vi "GD Status.vi"() -> (1 "Error":T1, 2 "Störung":bool, 3 "Status":string)   [LabVIEW 2020, in "EPA 1065.lvlib" / "HovaCAL Interference verificaton.lvlib"]
uses:
  HovaCAL Interference verificaton.lvlib
  Linearisierung V2/Gasteiler/AK-Komm Gasteiler/Aktionen AK Komm.ctl
  Linearisierung V2/Gasteiler/AK-Komm Gasteiler/AK Komm Gasteiler.lvlib
  Linearisierung V2/Aktion FGV Stoerungen sammeln und auswerten.ctl
  Linearisierung V2/Linearisierung v2.lvlib
  Linearisierung V2/Gasteiler/AK-Komm Gasteiler/Alter Gasteiler/Aktionen AK Komm_ALT.ctl
  Linearisierung V2/Gasteiler/AK-Komm Gasteiler/Alter Gasteiler/Alter Gasteiler.lvlib
  Linearisierung V2/Gasteiler/Horiba/Aktion Befehl.ctl
  Linearisierung V2/Gasteiler/Horiba/Horiba GDC.lvlib
  Linearisierung V2/Gasteiler/HovaCAL_Interface/Kommunikation/Aktion_FGV_HovaCAL_Interface_Kommandos.ctl
  Linearisierung V2/Gasteiler/HovaCAL_Interface/Kommunikation/Kommunikation.lvlib
  Linearisierung V2/Gasteiler/Aktionen FGV Gasteiler Daten.ctl
  Linearisierung V2/Gasteiler/Gasteiler.lvlib
  Linearisierung V2/Gasteiler/Gasteiler Fehler.ctl
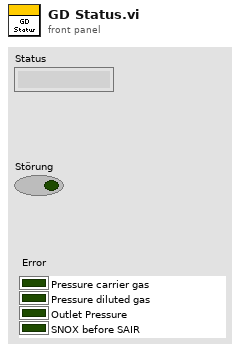
[diagram p1: front panel]
types:
  T1 = typedef "Linearisierung v2.lvlib/Gasteiler.lvlib/Gasteiler Fehler.ctl" = cluster{"Pressure carrier gas":bool, "Pressure diluted gas":bool, "Outlet Pressure":bool, "SNOX before SAIR":bool}
  T2 = typedef "Linearisierung v2.lvlib/Gasteiler.lvlib/Aktionen FGV Gasteiler Daten.ctl" = enum16{"lesen", "Gasteiler Daten", "Seriellen Param.", "MB-Endwert", "laden", "speichern", "Anforderung", "TCP", "Aufzeichnung Start"}
  T3 = typedef "Linearisierung v2.lvlib/GasteilerType.ctl" = u16
  T4 = typedef "Linearisierung v2.lvlib/Aktion FGV Stoerungen sammeln und auswerten.ctl" = enum16{"init", "lesen", "error", "prüfen", "reset error", "abbrechen", "fortsetzen", "neustart", "Bedientasten reset"}
  T5 = typedef "Linearisierung v2.lvlib/Gasteiler.lvlib/AK Komm Gasteiler.lvlib/Aktionen AK Komm.ctl" = enum16{"lesen", "initialisieren", "beenden", "Status", "SMAN", "SREM", "STBY", "ASTF", "ASTZ", "SLST", "AGAT", "EGAK", "AGAK", "AKAK", "ADRU", "SKOP", "SVSA", "SVSZ", "SONO", "SAIR", "SNOX", "ANOX", "SSPL", "SRUC", "SLIN", "ALST", "ETYP", "SVIO", "LCYL", "CCYL", "DCYL", "SCYL", "GCYL", "DRGV", "DRDC"}
  T6 = typedef "Linearisierung v2.lvlib/Gasteiler.lvlib/AK Komm Gasteiler.lvlib/Alter Gasteiler.lvlib/Aktionen AK Komm_ALT.ctl" = enum16{"lesen", "initialisieren", "beenden", "SRES", "STBY", "SREM", "SMAN", "SLIN", "SLCH", "SLST", "SSPL", "AGAT", "ALST", "ASTZ", "ASTF", "AGAK", "EGAK"}
  T7 = typedef "Linearisierung v2.lvlib/Gasteiler.lvlib/Horiba GDC.lvlib/Aktion Befehl.ctl" = enum16{"lesen", "initialisieren", "Beenden", "Standby", "GD/CC", "Info", "Flow", "Alarm", "GD parameter", "GD point", "Durchfluss", "Spuelen1", "Spuelen1 On", "Spuelen1Off", "Spuelen2", "Ventil-Abfrage", "Reset"}
  T8 = typedef "Linearisierung v2.lvlib/Gasteiler.lvlib/HovaCAL_Interface.lvlib/Kommunikation.lvlib/Aktion_FGV_HovaCAL_Interface_Kommandos.ctl" = enum16{"lesen", "verarbeiten", "hinzufügen", "on top", "init", "sammeln", "freigeben", "connected"}
  T9 = typedef "Linearisierung v2.lvlib/LIN ErrorCluster.ctl" = cluster{"Störung Kommunikation":bool, "Pressure carrier gas":bool, "Pressure diluted gas":bool, "Outlet Pressure":bool, "SNOX before SAIR":bool, "Störung Gasteiler":bool}
  T10 = cluster{"Pressure carrier gas":bool, "Pressure diluted gas":bool, "Outlet Pressure":bool, bool}
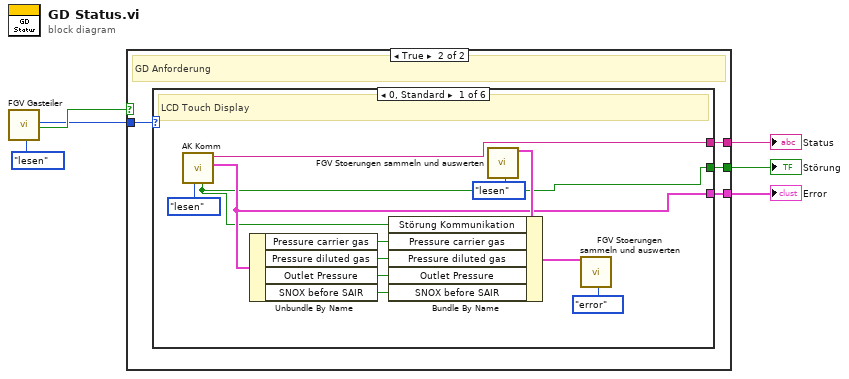
[diagram p0: block diagram]
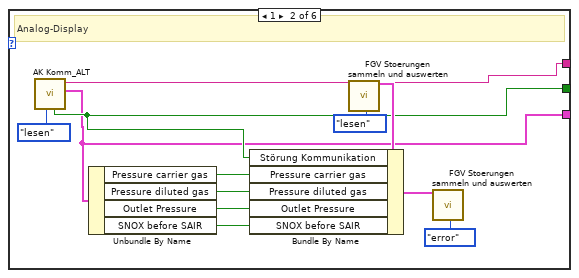
[diagram p3: hidden frame]
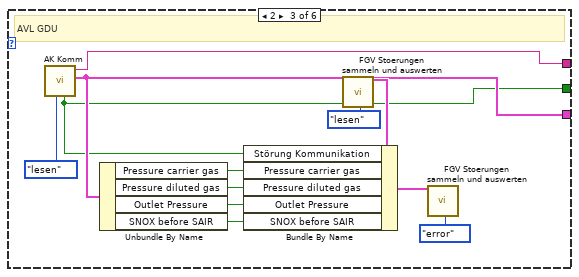
[diagram p4: hidden frame]
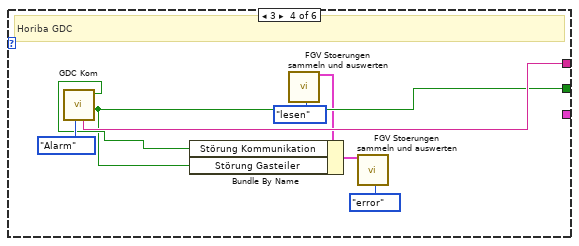
[diagram p5: hidden frame]
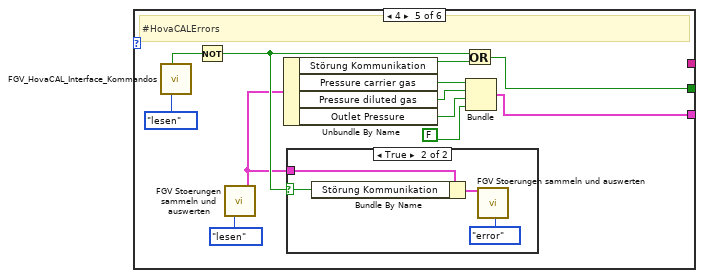
[diagram p6: hidden frame]
diagram:
  n1 = call "FGV Gasteiler.vi"("Aktionen"=Aktionen_FGV_Gasteiler_Daten."lesen") -> ("Gasteiler Type"=w2:T3, "Anforderung"=w3:bool)  [unwired: 11 in, 6 out]
  n2 = case shown="True" w3 {
    tunnel: w2 -> [_ w10]
    tunnel: [_ w9] -> w4
    tunnel: [_ w8] -> w5
    tunnel: [_ w7] -> w6
    frame False {
    }
    frame True {
      # "GD Anforderung"
      n3 = case shown="0, Standard" w10 {
        tunnel: [w12 w23 w37 _ w56 _] -> w9
        tunnel: [w11 w24 w36 w48 w55 _] -> w8
        tunnel: [w13 w25 w35 w50 _ _] -> w7
        frame 0, Default {
          # "LCD Touch Display"
          n4 = call "AK Komm.vi"("Aktionen"=Aktionen_AK_Komm."lesen") -> ("Error"=w12:T1, "Status"=w13:string, "Störung Kommunikation"=w11:bool)  [unwired: 4 in, 4 out]
          n5 = Unbundle By Name(w12) -> ("Pressure carrier gas"=w18:bool, "Pressure diluted gas"=w17:bool, "Outlet Pressure"=w16:bool, "SNOX before SAIR"=w15:bool)
          n6 = call "FGV Stoerungen sammeln und auswerten.vi"("Aktion"=Aktion_FGV_Stoerungen_sammeln_und_auswerten."lesen") -> ("Errors"=w19:T9)  [unwired: 12 in, 6 out]
          n7 = Bundle By Name(cluster=w19, "Störung Kommunikation"=w11, "Pressure carrier gas"=w18, "Pressure diluted gas"=w17, "Outlet Pressure"=w16, "SNOX before SAIR"=w15) -> (w14:T9)
          n8 = call "FGV Stoerungen sammeln und auswerten.vi"("Errors"=w14, "Aktion"=Aktion_FGV_Stoerungen_sammeln_und_auswerten."error") -> ()  [unwired: 11 in, 7 out]
        }
        frame 1 {
          # "Analog-Display"
          n9 = call "AK Komm_ALT.vi"("Aktionen_ALT"=Aktionen_AK_Komm_ALT."lesen") -> ("Error"=w23:T1, "Status"=w25:string, "Störung Kommunikation"=w24:bool)  [unwired: 6 in, 2 out]
          n10 = Unbundle By Name(w23) -> ("Pressure carrier gas"=w30:bool, "Pressure diluted gas"=w29:bool, "Outlet Pressure"=w28:bool, "SNOX before SAIR"=w27:bool)
          n11 = call "FGV Stoerungen sammeln und auswerten.vi"("Aktion"=Aktion_FGV_Stoerungen_sammeln_und_auswerten."lesen") -> ("Errors"=w31:T9)  [unwired: 12 in, 6 out]
          n12 = Bundle By Name(cluster=w31, "Störung Kommunikation"=w24, "Pressure carrier gas"=w30, "Pressure diluted gas"=w29, "Outlet Pressure"=w28, "SNOX before SAIR"=w27) -> (w26:T9)
          n13 = call "FGV Stoerungen sammeln und auswerten.vi"("Errors"=w26, "Aktion"=Aktion_FGV_Stoerungen_sammeln_und_auswerten."error") -> ()  [unwired: 11 in, 7 out]
        }
        frame 2 {
          # "AVL GDU"
          n14 = call "AK Komm.vi"("Aktionen"=Aktionen_AK_Komm."lesen") -> ("Error"=w37:T1, "Status"=w35:string, "Störung Kommunikation"=w36:bool)  [unwired: 4 in, 4 out]
          n15 = Unbundle By Name(w37) -> ("Pressure carrier gas"=w42:bool, "Pressure diluted gas"=w41:bool, "Outlet Pressure"=w40:bool, "SNOX before SAIR"=w39:bool)
          n16 = call "FGV Stoerungen sammeln und auswerten.vi"("Aktion"=Aktion_FGV_Stoerungen_sammeln_und_auswerten."lesen") -> ("Errors"=w43:T9)  [unwired: 12 in, 6 out]
          n17 = Bundle By Name(cluster=w43, "Störung Kommunikation"=w36, "Pressure carrier gas"=w42, "Pressure diluted gas"=w41, "Outlet Pressure"=w40, "SNOX before SAIR"=w39) -> (w38:T9)
          n18 = call "FGV Stoerungen sammeln und auswerten.vi"("Errors"=w38, "Aktion"=Aktion_FGV_Stoerungen_sammeln_und_auswerten."error") -> ()  [unwired: 11 in, 7 out]
        }
        frame 3 {
          # "Horiba GDC"
          n19 = call "GDC Kom.vi"("Befehl"=Aktion_Befehl."Alarm") -> ("Status (alarm)"=w48:bool, "Fehler"=w49:bool, "Status"=w50:string)  [unwired: 4 in, 4 out]
          n20 = call "FGV Stoerungen sammeln und auswerten.vi"("Aktion"=Aktion_FGV_Stoerungen_sammeln_und_auswerten."lesen") -> ("Errors"=w47:T9)  [unwired: 12 in, 6 out]
          n21 = Bundle By Name(cluster=w47, "Störung Kommunikation"=w49, "Störung Gasteiler"=w48) -> (w51:T9)
          n22 = call "FGV Stoerungen sammeln und auswerten.vi"("Errors"=w51, "Aktion"=Aktion_FGV_Stoerungen_sammeln_und_auswerten."error") -> ()  [unwired: 11 in, 7 out]
        }
        frame 4 {
          # "#HovaCALErrors"
          n23 = call "FGV_HovaCAL_Interface_Kommandos.vi"("Aktion"=Aktion_FGV_HovaCAL_Interface_Kommandos."lesen") -> ("connected out ?"=w58:bool)  [unwired: 4 in, 5 out]
          n24 = Not(x=w58) -> (.not. x?=w59:bool)
          n25 = call "FGV Stoerungen sammeln und auswerten.vi"("Aktion"=Aktion_FGV_Stoerungen_sammeln_und_auswerten."lesen") -> ("Errors for AutoSPAN"=w57:T9)  [unwired: 12 in, 6 out]
          n26 = Unbundle By Name(w57) -> ("Störung Kommunikation"=w65:bool, "Pressure carrier gas"=w64:bool, "Pressure diluted gas"=w63:bool, "Outlet Pressure"=w62:bool)
          n27 = case shown="True" w59 {
            selector: w59 -> [_ w68]
            tunnel: w57 -> [_ w67]
            frame False {
            }
            frame True {
              n28 = Bundle By Name(cluster=w67, "Störung Kommunikation"=w68) -> (w69:T9)
              n29 = call "FGV Stoerungen sammeln und auswerten.vi"("Errors"=w69, "Aktion"=Aktion_FGV_Stoerungen_sammeln_und_auswerten."error") -> ()  [unwired: 11 in, 7 out]
            }
          }
          n30 = Or(x=w59, y=w65) -> (x .or. y?=w55:bool)
          n31 = Bundle("Pressure carrier gas"=w64, "Pressure diluted gas"=w63, "Outlet Pressure"=w62, FALSE) -> (w56:T10)  [unwired: 1 in]
        }
        frame 5 {
          # "manuell"
        }
      }
    }
  }
  "Status" <- w6
  "Störung" <- w5
  "Error" <- w4
